vi "Cycle.vi"(8 "error in (no error)":errorcluster, 11 "PassiveExperiment In":refnum<class "PassiveExperiment.lvclass">) -> (0 "error out":errorcluster, 3 "PassiveExperiment Out":refnum<class "PassiveExperiment.lvclass">)   [LabVIEW 2010, in "PassiveExperiment.lvclass"]
uses:
  PassiveExperiment.lvclass
  MatlabExperiment/MatlabExperiment.lvclass
panel:
  out "ExperimentStats":T1
  in  "FixationRadius":dbl
  in  "Correct Reward Time":dbl
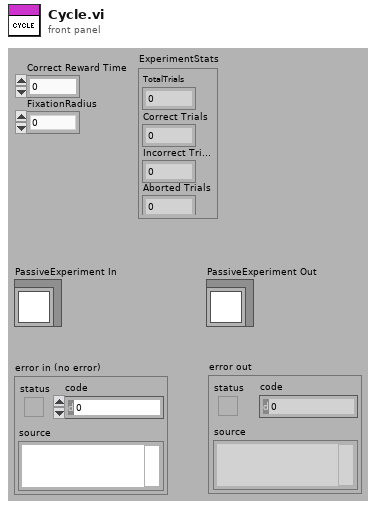
[diagram p1: front panel]
types:
  T1 = cluster{"TotalTrials":dbl, "Correct Trials":dbl, "Incorrect Trials":dbl, "Aborted Trials":dbl}
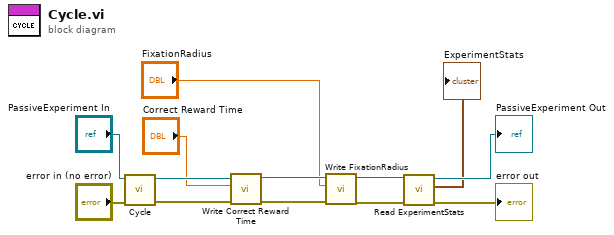
[diagram p0: block diagram]
diagram:
  n1 = call-parent "Cycle.vi"("error in (no error)"="error in (no error)", "MatlabExperiment In"="PassiveExperiment In") -> ("error out"=w10:errorcluster, "MatlabExperiment Out"=w11:refnum<class "PassiveExperiment.lvclass">)  [unwired: 8 in]
  n2 = call-dynamic "Write Correct Reward Time.vi"("error in (no error)"=w10, "Correct Reward Time"="Correct Reward Time", "MatlabExperiment in"=w11) -> ("error out"=w8:errorcluster, "MatlabExperiment out"=w9:refnum<class "PassiveExperiment.lvclass">)  [unwired: 7 in]
  n3 = call-dynamic "Write FixationRadius.vi"("error in (no error)"=w8, "FixationRadius"="FixationRadius", "MatlabExperiment in"=w9) -> ("error out"=w4:errorcluster, "MatlabExperiment out"=w5:refnum<class "PassiveExperiment.lvclass">)  [unwired: 7 in]
  n4 = call-dynamic "Read ExperimentStats.vi"("error in (no error)"=w4, "TrialBasedExperiment in"=w5) -> ("error out"=→"error out":errorcluster, "ExperimentStats"=→"ExperimentStats":T1, "TrialBasedExperiment out"=→"PassiveExperiment Out":refnum<class "PassiveExperiment.lvclass">)  [unwired: 7 in]
